vi "From Variant.vi"(8 "Error In":errorcluster, 10 "Variant":variant, 11 "2D Int In":refnum<class "2D Int.lvclass">) -> (0 "Error Out":errorcluster, 3 "2D Int Out":refnum<class "2D Int.lvclass">)   [LabVIEW 2020, in "NI_VIAnCFGDataStructure.lvlib" / "2D Int.lvclass"]
doc: "Dynamic dispatch interface for conversion of variant LV data to Tree Data classes."
uses:
  <vilib>/addons/analyzer/VIAnCFGDataStructure/Data Types/2D Int/2D Int.lvclass
  <vilib>/addons/analyzer/VIAnCFGDataStructure/Data Types/2D Int/2D Int.lvclass/2D Int.ctl
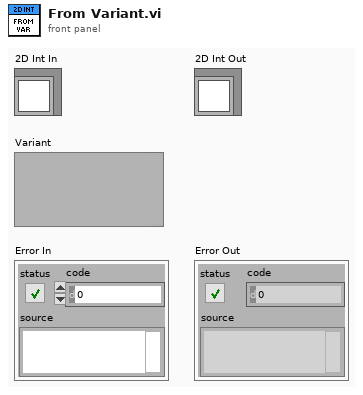
[diagram p1: front panel]
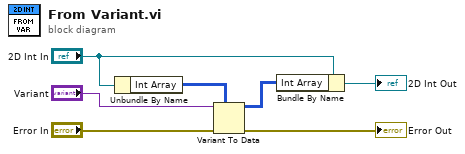
[diagram p0: block diagram]
diagram:
  n1 = Unbundle By Name("2D Int In") -> ("Int Array"=w6:i64[][])
  n2 = Variant To Data(error in="Error In", type=w6, Variant="Variant") -> (data=w4:i64[][], error out=→"Error Out":errorcluster)
  n3 = Bundle By Name(cluster="2D Int In", "Int Array"=w4) -> (→"2D Int Out":refnum<class "2D Int.lvclass">)
